vi "AttrMap-SetValue-CORE.vi"(8 "error in (no error)":errorcluster, 9 "Value":variant, 10 "Key":string, 11 "AttrMap in":T1) -> (0 "error out":errorcluster, 3 "AttrMap out":T1, 4 "OrgKey String":string)   [LabVIEW 2019, in "lv-apt-json-file.lvlib"]
uses:
  lv-apt-json-file.lvlib
  Typedef/Def-AttrMap.ctl
  6e91e2cf-a420-477d-bf86-627245081caf.vi
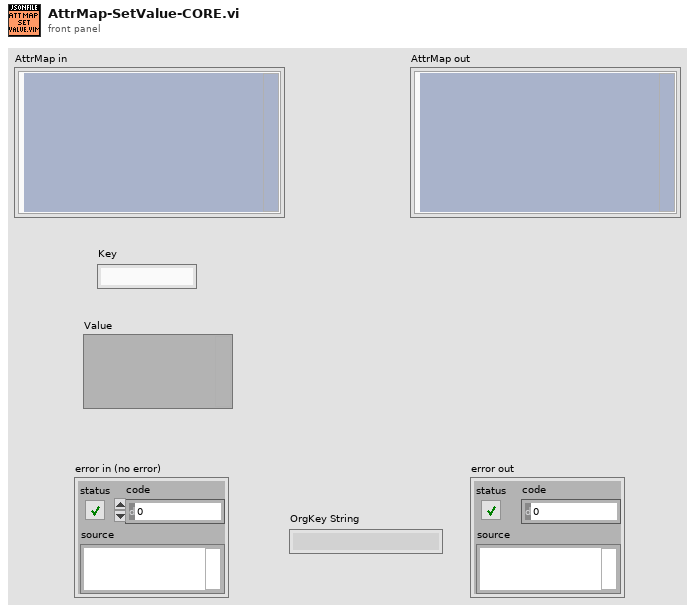
[diagram p1: front panel]
types:
  T1 = typedef "lv-apt-json-file.lvlib/Def-AttrMap.ctl" = cluster{"Map":variant}
  T2 = typedef "lv-apt-json-file.lvlib/Def-AttrMap -- NameMap.ctl" = map{string, string}
  T3 = typedef "Type Descriptor Enumeration__ogtk.ctl" = enum8{"<Null>", "I8", "I16", "I32", "I64", "U8", "U16", "U32", "U64", "SGL", "DBL", "EXT", "CSG", "CDB", "CXT", "0x0F", "0x10", "0x11", "0x12", "0x13", "0x14", "Enum U8", "Enum U16", "Enum U32", "Enum U64", "SGL PQ", "DBL PQ", "EXT PQ", "CSG PQ", "CDB PQ", "CXT PQ", "0x1F", "0x20", "Boolean", "0x22", "0x23", "0x24", "0x25", "0x26", "0x27", "0x28", "0x29", "0x2A", "0x2B", "0x2C", "0x2D", "0x2E", "0x2F", "String", "0x31", "Path", "Pict", "0x34", "0x35", "0x36", "DAQ", "0x38", "0x39", "0x3A", "0x3B", "0x3C", "0x3D", "0x3E", "0x3F", "Array", "0x41", "0x42", "0x43", "0x44", "0x45", "0x46", "0x47", "0x48", "0x49", "0x4A", "0x4B", "0x4C", "0x4D", "0x4E", "0x4F", "Cluster", "0x51", "0x52", "Variant", "Waveform", "0x55", "0x56", "0x57", "0x58", "0x59", "0x5A", "0x5B", "0x5C", "0x5D", "0x5E", "0x5F", "0x60", "0x61", "0x62", "0x63", "0x64", "0x65", "0x66", "0x67", "0x68", "0x69", "0x6A", "0x6B", "0x6C", "0x6D", "0x6E", "0x6F", "Refnum"}
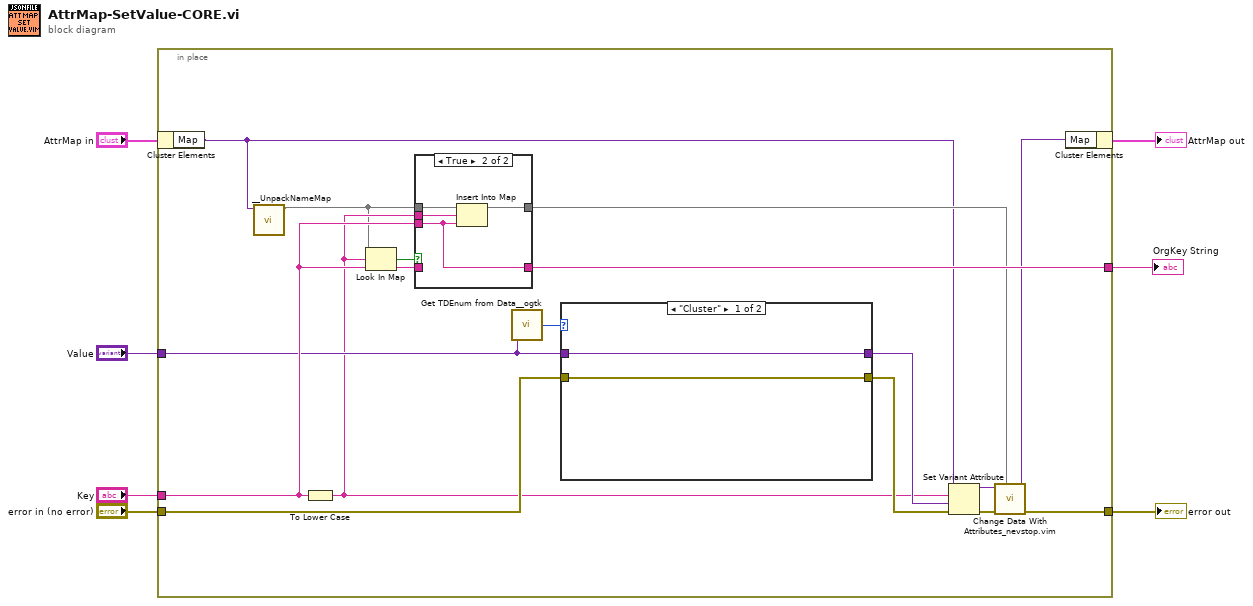
[diagram p0: block diagram]
diagram:
  n1 = in-place {
    in-place-border: [w24] -> w7
    in-place-border: "error in (no error)" -> [w23]
    in-place-border: "Key" -> [w22]
    in-place-border: "Value" -> [w21]
    in-place-border: [w20] -> w3
    n2 = in-place-cluster #1("AttrMap in") -> ("Map"=w9:variant)
    n3 = call "__UnpackNameMap.vi"("Map"=w9) -> ("NameMap"=w8:T2)  [unwired: 10 in]
    n4 = To Lower Case(string=w22) -> (all lower case string=w13:string)
    n5 = Look In Map(map=w8, key=w13, default value=w22) -> (key not found?=w12:bool, value=w11:string)
    n6 = case shown="True" w12 {
      tunnel: w8 -> [w26 w30]
      tunnel: [w26 w29] -> w14
      tunnel: w13 -> [_ w28]
      tunnel: w22 -> [_ w27]
      tunnel: w11 -> [w25 _]
      tunnel: [w25 w27] -> w20
      frame False {
      }
      frame True {
        n7 = Insert Into Map(map in=w30, key=w28, value=w27) -> (map out=w29:T2)  [unwired: 2 out]
      }
    }
    n8 = call <userlib>:"Get TDEnum from Data__ogtk.vi"("Data"=w21) -> ("Type Descriptor Enumeration"=w17:T3)  [unwired: 4 in]
    n9 = case shown="\"Cluster\"" w17 {
      tunnel: w21 -> [w32 w33]
      tunnel: w23 -> [w31 w34]
      tunnel: [w31 w34] -> w19
      tunnel: [w32 w33] -> w18
      frame "Cluster" {
      }
      frame Default {
      }
    }
    n10 = Set Variant Attribute(Variant=w9, name=w13, value=w18, error in=w19) -> (Variant out=w16:variant, error out=w15:errorcluster)  [unwired: 1 out]
    n11 = call "Change Data With Attributes_nevstop.vim"("Data"=w14, "error in (no error)"=w15, "Variant in"=w16) -> ("error out"=w24:errorcluster, "Variant out"=w10:variant)  [unwired: 7 in]
    n12 = in-place-cluster #1("Map"=w10) -> (→"AttrMap out":T1)
  }
  "error out" <- w7
  "OrgKey String" <- w3
